vi "libssh2_channel_direct_tcpip_ex.vi"(4 "sport":i32, 6 "shost":string, 8 "error in (no error)":errorcluster, 9 "port":i32, 10 "host":string, 11 "session":T2) -> (0 "error out":errorcluster, 3 "channel":T1)   [LabVIEW 2013, in "libssh2.lvlib"]
doc: "Create a channel to tunnel a TCP connection from a local port to a target host through an SSH session. Communication to the SSH server remains encrypted. Communication from the SSH server to the target host happens in clear text."
uses:
  libssh2.lvlib
  Session Refnum.ctl
  Channel Refnum.ctl
  Not A Session.vi
  <vilib>/Utility/error.llb/Error Cluster From Error Code.vi
  Global Settings.vi
  Read Session Refnum.vi
  <vilib>/Utility/semaphor.llb/Acquire Semaphore.vi
  <vilib>/Utility/semaphor.llb/Release Semaphore.vi
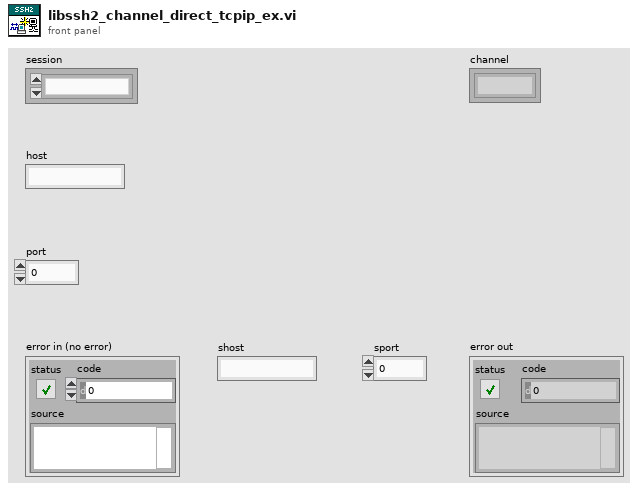
[diagram p1: front panel]
types:
  T1 = typedef "libssh2.lvlib/Channel Refnum.ctl" = refnum<k1>
  T2 = typedef "libssh2.lvlib/Session Refnum.ctl" = refnum<k1>
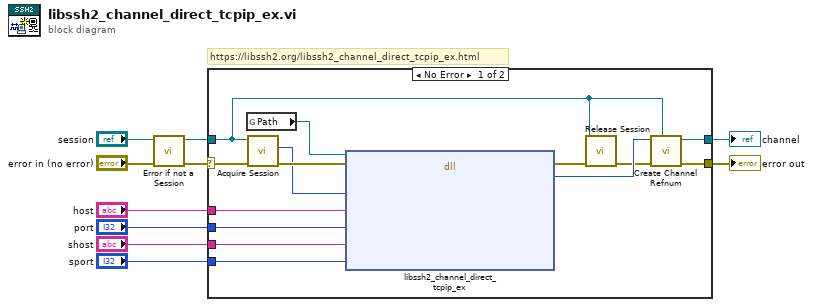
[diagram p0: block diagram]
diagram:
  # "https://libssh2.org/libssh2_channel_direct_tcpip_ex.html"
  n1 = call "Error if not a Session.vi"("error in (no error)"="error in (no error)", "session"="session") -> ("error out"=w3:errorcluster, "session out"=w1:T2)  [unwired: 8 in]
  n2 = case shown="No Error" w3 {
    selector: w3 -> [w14 w25]
    tunnel: "host" -> [w23 _]
    tunnel: "port" -> [w22 _]
    tunnel: "shost" -> [w21 _]
    tunnel: "sport" -> [w20 _]
    tunnel: w1 -> [w11 _]
    tunnel: [w17 w25] -> w6
    tunnel: [w15 _] -> w5
    frame No Error {
      n3 = global read "Global Settings.vi" "Path"() -> (w13:path)
      n4 = call "Acquire Session.vi"("error in (no error)"=w14, "session"=w11) -> ("error out"=w19:errorcluster, "LIBSSH2_SESSION*"=w18:u64)  [unwired: 7 in, 1 out]
      n5 = dll-call lib="?" fn="libssh2_channel_direct_tcpip_ex"(path in=w13, error in=w19, "session"=w18, "host"=w23, "port"=w22, "shost"=w21, "sport"=w20) -> (error out=w24:errorcluster, "return value"=w16:u64)  [unwired: 6 in, 1 out]
      n6 = call "Release Session.vi"("error in (no error)"=w24, "session"=w11) -> ("error out"=w12:errorcluster)  [unwired: 9 in]
      n7 = call "Create Channel Refnum.vi"("session"=w11, "error in (no error)"=w12, "LIBSSH2_CHANNEL*"=w16) -> ("error out"=w17:errorcluster, "channel"=w15:T1)  [unwired: 7 in]
    }
    frame Error {
    }
  }
  "error out" <- w6
  "channel" <- w5
